vi "Project.vi"() -> ()   [LabVIEW 2014]
uses:
  <vilib>/express/express shared/transition.llb/Dynamic To Waveform Array.vi
  <vilib>/express/express arith-compare/Formula/Block/exnFormulaBlock how many pts in the wave.vi
  <vilib>/express/express shared/ex_Modify Signal Name.vi
  <vilib>/express/express shared/transition.llb/Waveform Array To Dynamic.vi
  <vilib>/express/express arith-compare/Formula/XNode/ExpressFormulaBlockNode.xnode
panel:
  out "P4 2":dbl
  out "P3":dbl
  out "P2":dbl
  out "P1":dbl
  out "Bottom":bool
  out "Right":bool
  out "Top_Left":bool
  out "Top":bool
  out "Meter 4":dbl(knob) scale=-10.0..10.0
  out "Meter 3":dbl(knob) scale=-10.0..10.0
  out "Meter 2":dbl(knob) scale=-10.0..10.0
  out "Meter":dbl(knob) scale=-10.0..10.0
  out "Waveform Graph 4":dynamicdata(graph)
  out "Waveform Graph 3":dynamicdata(graph)
  out "Waveform Graph 2":dynamicdata(graph)
  out "Waveform Graph":dynamicdata(graph)
  in  "STOP":bool
  out "V4":dbl
  out "V3":dbl
  out "V2":dbl
  out "V1":dbl
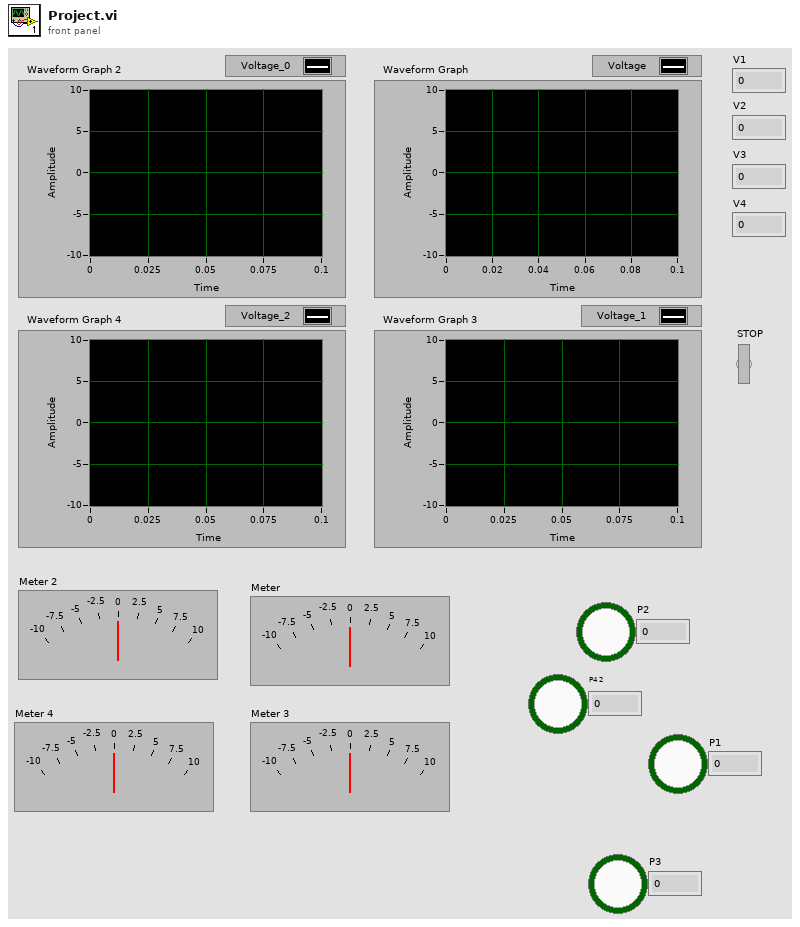
[diagram p1: front panel]
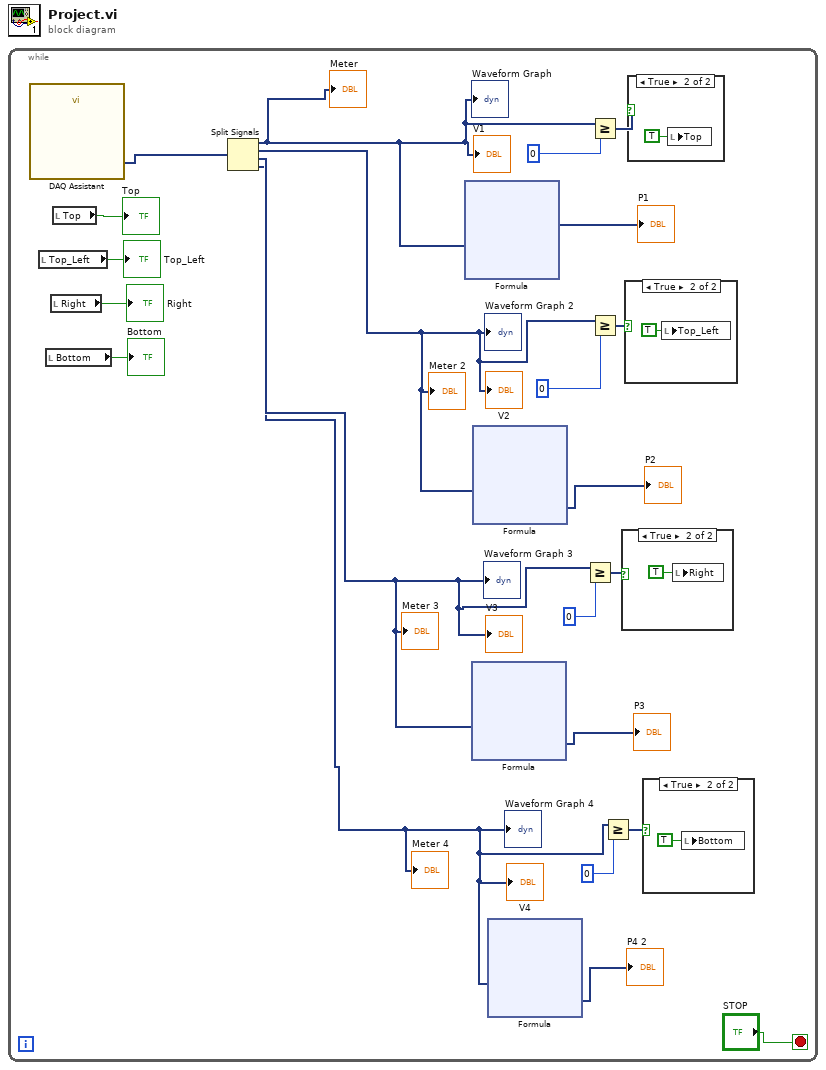
[diagram p0: block diagram]
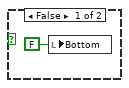
[diagram p2: hidden frame]
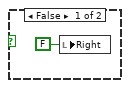
[diagram p3: hidden frame]
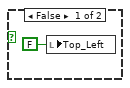
[diagram p4: hidden frame]
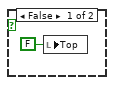
[diagram p5: hidden frame]
diagram:
  n1 = while {
    stop <- "STOP" stop-if-true
    n2 = call "DAQ Assistant"() -> ("data"=w9:dynamicdata)  [unwired: 17 in, 2 out]
    n3 = local read "Top_Left"() -> (→"Top_Left":bool)
    n4 = local read "Bottom"() -> (→"Bottom":bool)
    n5 = local read "Right"() -> (→"Right":bool)
    n6 = local read "Top"() -> (→"Top":bool)
    n7 = Split Signals(w9) -> (w7:dynamicdata, w6:dynamicdata, w4:dynamicdata, w1:dynamicdata)  [unwired: 4 in]
    "V3" <- w4
    "V1" <- w7
    "V2" <- w6
    "V4" <- w1
    "Waveform Graph" <- w7
    "Waveform Graph 2" <- w6
    "Waveform Graph 3" <- w4
    "Waveform Graph 4" <- w1
    "Meter" <- w7
    "Meter 2" <- w6
    "Meter 3" <- w4
    "Meter 4" <- w1
    n8 = xnode "Formula"("X1"=w7) -> ("Result"=→"P1":dynamicdata)  [unwired: 1 in, 1 out]
    n9 = xnode "Formula"("X1"=w4) -> ("Result"=→"P3":dynamicdata)  [unwired: 1 in, 1 out]
    n10 = xnode "Formula"("X1"=w6) -> ("Result"=→"P2":dynamicdata)  [unwired: 1 in, 1 out]
    n11 = xnode "Formula"("X1"=w1) -> ("Result"=→"P4 2":dynamicdata)  [unwired: 1 in, 1 out]
    n12 = Greater Or Equal?(x=w4, y=0) -> (x >= y?=w12:dynamicdata)
    n13 = Greater Or Equal?(x=w7, y=0) -> (x >= y?=w20:dynamicdata)
    n14 = Greater Or Equal?(x=w6, y=0) -> (x >= y?=w18:dynamicdata)
    n15 = Greater Or Equal?(x=w1, y=0) -> (x >= y?=w10:dynamicdata)
    n16 = case shown="True" w12 {
      frame False {
        n17 = local write "Right"(FALSE ("Right")) -> ()
      }
      frame True {
        n18 = local write "Right"(TRUE ("Right")) -> ()
      }
    }
    n19 = case shown="True" w18 {
      frame False {
        n20 = local write "Top_Left"(FALSE ("Top_Left")) -> ()
      }
      frame True {
        n21 = local write "Top_Left"(TRUE ("Top_Left")) -> ()
      }
    }
    n22 = case shown="True" w20 {
      frame False {
        n23 = local write "Top"(FALSE ("top")) -> ()
      }
      frame True {
        n24 = local write "Top"(TRUE ("top")) -> ()
      }
    }
    n25 = case shown="True" w10 {
      frame False {
        n26 = local write "Bottom"(FALSE ("Bottom")) -> ()
      }
      frame True {
        n27 = local write "Bottom"(TRUE ("Bottom")) -> ()
      }
    }
  }
